vi "5.10 Probabalistic Alg Sub 1.vi"(2 "Input Data":u8[][](array[numeric])) -> (5 "Pixelsum":i32, 6 "StdDev":dbl[](array[numeric]), 7 "EigenVector1":dbl[](array[numeric]), 8 "Sizes":i32[](array[numeric]), 9 "EigenVector2":dbl[](array[numeric]), 10 "mean vector":dbl[](array[numeric]))   [LabVIEW 2011]
uses:
  <vilib>/Analysis/7linalg.llb/Eigenvalue and Vectors Output Option.ctl
  <vilib>/Analysis/7linalg.llb/Real Eigenvalues and Vectors.vi
  <vilib>/Analysis/Matrix/Numeric/Complex/Complex To Cartesian - CM.vi
  <vilib>/Analysis/NI_AALPro.lvlib
  <vilib>/Analysis/Matrix/NI_Matrix.lvlib
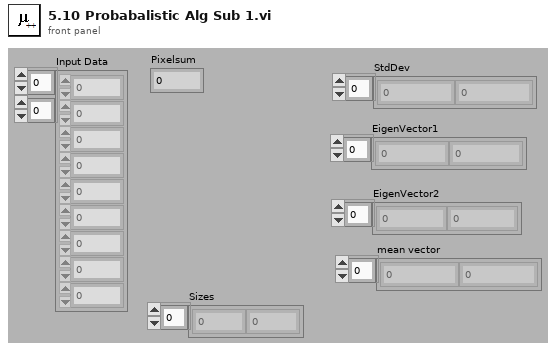
[diagram p1: front panel]
types:
  T1 = typedef "NI_AALPro.lvlib/Eigenvalue and Vectors Output Option.ctl" = i32
  T2 = typedef "NI_Matrix.lvlib/RealMatrix.ctl" = dbl[][]
  T3 = typedef "NI_Matrix.lvlib/ComplexMatrix.ctl" = cdb[][]
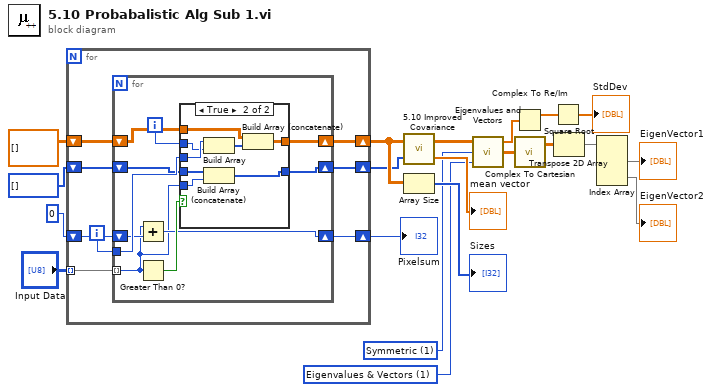
[diagram p0: block diagram]
diagram:
  w9 = T1 1 items=["Eigenvalues", "Eigenvalues & Vectors"] ("output option")
  w8 = 1 items=["General", "Symmetric"] ("matrix type")
  n1 = for {
    tunnel: "Input Data" -> [w28] mode=indexing
    shift-right: [w25] -> w11
    shift-left: dbl[][] [] ("X 2") -> [w27]
    shift-right: [w23] -> w20
    shift-left: 0 -> [w24]
    shift-right: [w21] -> w1
    shift-left: u8[] [] ("X 2") -> [w22]
    i -> [w26]
    n2 = for {
      tunnel: w28 -> [w30] mode=indexing
      shift-right: [w35] -> w25
      shift-left: w27 -> [w36]
      tunnel: w26 -> [w38]
      shift-right: [w32] -> w23
      shift-left: w24 -> [w33]
      shift-right: [w29] -> w21
      shift-left: w22 -> [w31]
      i -> [w37]
      n3 = Add(x=w30, y=w33) -> (x+y=w32:i32)
      n4 = Greater Than 0?(x=w30) -> (x > 0?=w34:bool)
      n5 = case shown="True" w34 {
        tunnel: w38 -> [_ w48]
        tunnel: w37 -> [_ w47]
        tunnel: w36 -> [w40 w46]
        tunnel: [w40 w44] -> w35
        tunnel: w31 -> [w39 w43]
        tunnel: [w39 w42] -> w29
        tunnel: w30 -> [_ w41]
        frame False {
        }
        frame True {
          n6 = Build Array(w48, w47) -> (w45:i32[])
          n7 = Build Array (concatenate)(w43, w41) -> (w42:u8[])
          n8 = Build Array (concatenate)(w46, w45) -> (w44:dbl[][])
        }
      }
    }
  }
  "Pixelsum" <- w20
  n9 = call "5.10 Improved Covariance.vi"("Scaling"=w1, "X"=w11) -> ("mean vector"=→"mean vector":dbl[], "covariance matrix V"=w7:T2)
  n10 = Array Size(array=w11) -> (size(s)=→"Sizes":i32[])
  n11 = call-poly <vilib>:"Eigenvalues and Vectors.vi"("output option"=w9, "matrix type"=w8, "Input Matrix"=w7) -> ("Eigenvectors"=w13:T3, "Eigenvalues"=w14:cdb[])  [unwired: 1 out]
  n12 = Complex To Re/Im ("Complex To Cartesian.vi")(x + iy=w14) -> (x=w15:dbl[])  [unwired: 1 out]
  n13 = call-poly <vilib>:"Complex To Cartesian.vi"("Complex Matrix R + Ii"=w13) -> ("Real Matrix R"=w5:T2)  [unwired: 1 out]
  n14 = Square Root(x=w15) -> (sqrt(x)=→"StdDev":dbl[])
  n15 = Transpose 2D Array(2D array=w5) -> (transposed array=w6:T2)
  n16 = Index Array(array=w6) -> (element #1=→"EigenVector1":dbl[], element #2=→"EigenVector2":dbl[])  [unwired: 4 in]
